vi "Reset.vi"(8 "error in (no error)":errorcluster caption="entrée d'erreur (pas d'erreur)", 11 "Class UART (Default) en entrée":refnum<class "Class UART (Default).lvclass">) -> (0 "error out":errorcluster caption="sortie d'erreur", 3 "Class UART (Default) en sortie":refnum<class "Class UART (Default).lvclass">)   [LabVIEW 2020, in "Library Instrument & Equipement.lvlib" / "Library UART.lvlib" / "Class UART (Default).lvclass"]
uses:
  Class UART (Default).lvclass
  Class UART (Default).lvclass/Class UART (Default).ctl
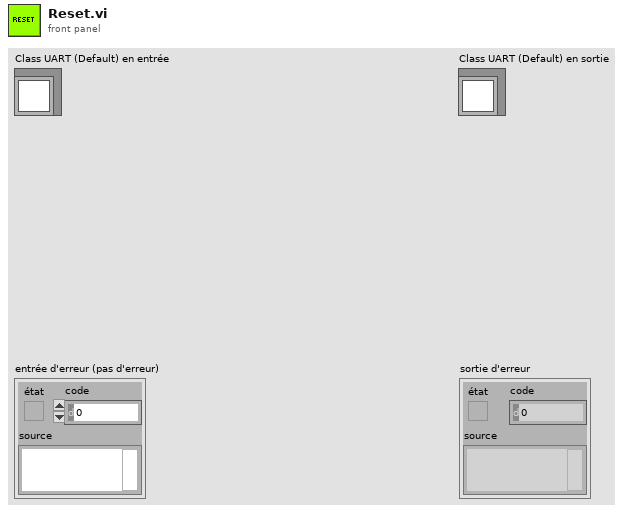
[diagram p1: front panel]
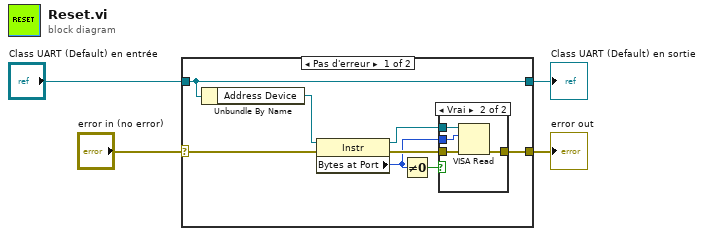
[diagram p0: block diagram]
diagram:
  n1 = case shown="Pas d'erreur" "error in (no error)" {
    selector: "error in (no error)" -> [w9 w19]
    tunnel: [w11 w19] -> w3
    tunnel: [w12 w18] -> w1
    tunnel: "Class UART (Default) en entrée" -> [w12 w18]
    frame No Error {
      n2 = Unbundle By Name(w12) -> ("Address Device"=w10:refnum<visa-resource-name>)
      n3 = property class="Instr"(reference=w10, error in=w9) -> (reference out=w7:refnum<visa-resource-name>, error out=w8:errorcluster, "Bytes at Port"=w6:u32)
      n4 = Not Equal To 0?(x=w6) -> (x != 0?=w5:bool)
      n5 = case shown="Vrai" w5 {
        tunnel: [w13 w17] -> w11
        tunnel: w6 -> [_ w16]
        tunnel: w8 -> [w13 w15]
        tunnel: w7 -> [_ w14]
        frame False {
        }
        frame True {
          n6 = VISA Read(VISA resource name=w14, byte count=w16, error in (no error)=w15) -> (error out=w17:errorcluster)  [unwired: 3 out]
        }
      }
    }
    frame Error {
    }
  }
  "error out" <- w3
  "Class UART (Default) en sortie" <- w1
